vi "Generate SBOM from VIPC.vi"() -> ()   [LabVIEW 2017]
uses:
  <vilib>/JKI/VIPM API/command-line/support/Library Contents Cluster_vipm_api.ctl
  <vilib>/JKI/VIPM API/VIPM API_vipm_api.lvlib
  VIP Support/VIP SBOM Support.lvlib
panel:
  in  "VIPC File Path":path
  out "SBOM":string[][](table)
  out "CSV SBOM":string
  out "Packages in VIPC":T1[](array[typedef])
  # "Retrieves package information from the specified VIPC file"
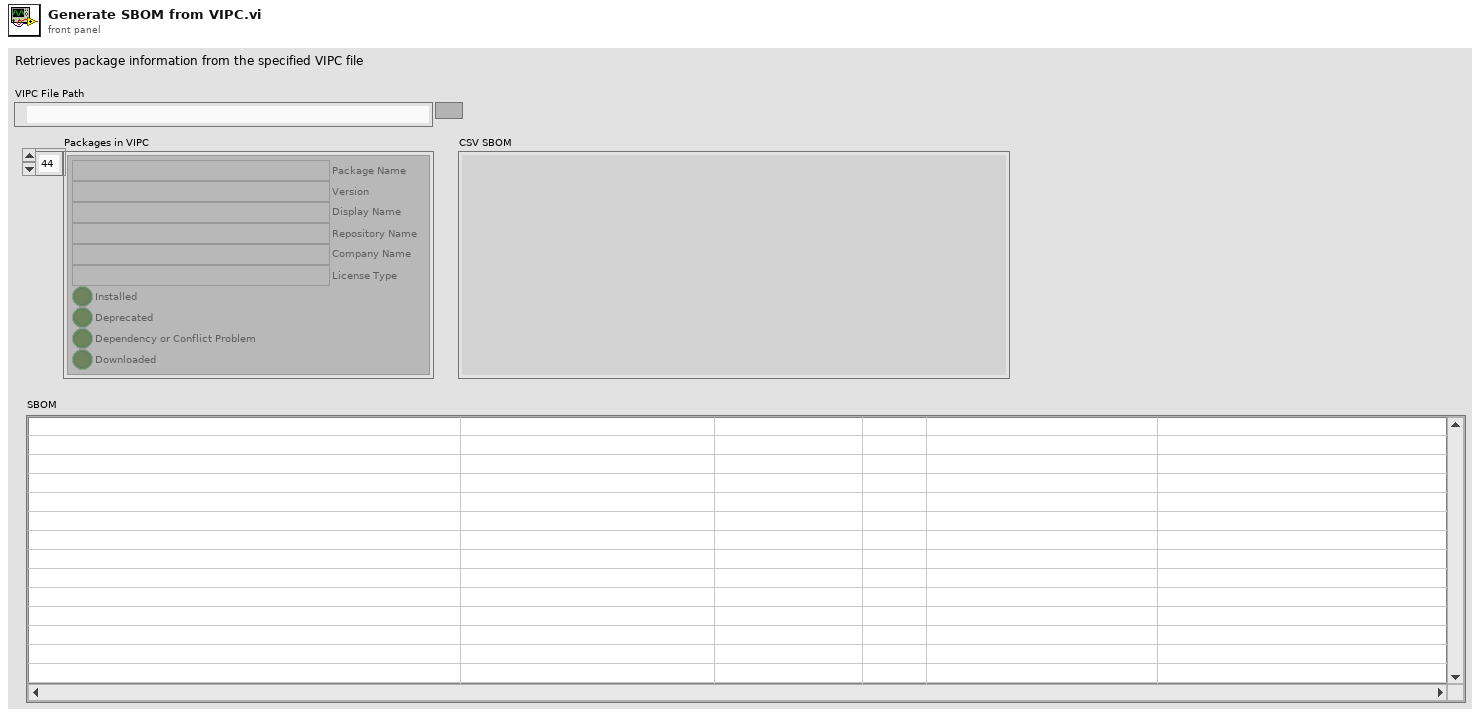
[diagram p1: front panel]
types:
  T1 = typedef "VIPM API_vipm_api.lvlib/Library Contents Cluster_vipm_api.ctl" = cluster{"Package Name":string, "Version":string, "Display Name":string, "Repository Name":string, "Company Name":string, "License Type":string, "Installed":bool, "Deprecated":bool, "Dependency or Conflict Problem":bool, "Downloaded":bool}
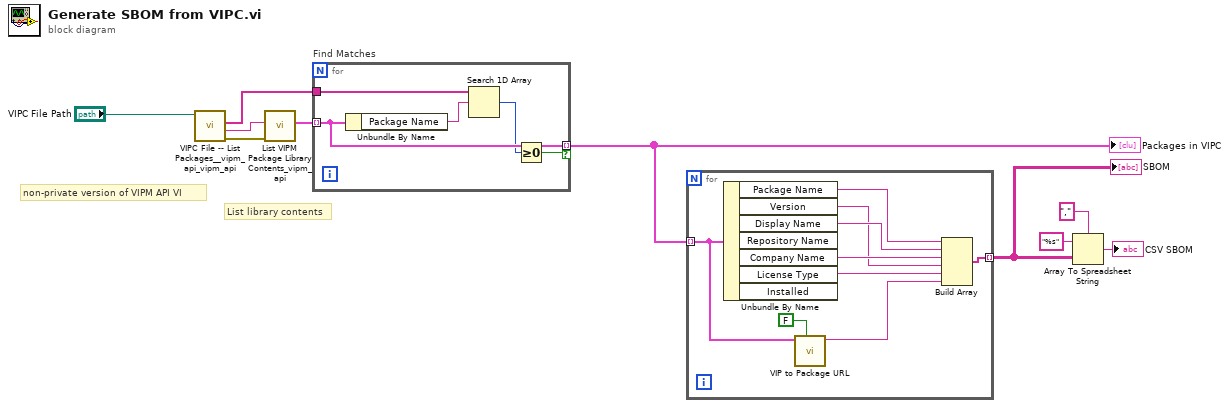
[diagram p0: block diagram]
diagram:
  # "List library contents"
  # "non-private version of VIPM API VI"
  n1 = call "VIPC File -- List Packages__vipm_api_vipm_api.vi"("VIPC File Path"="VIPC File Path") -> ("error out"=w3:errorcluster, "VIPC LabVIEW Version"=w1:string, "Package List"=w2:string[])  [unwired: 7 in, 1 out]
  n2 = call <vilib>:"List VIPM Package Library Contents_vipm_api.vi"("error in (no error)"=w3, "LabVIEW Version"=w1) -> ("Library Contents []"=w5:T1[])  [unwired: 8 in, 1 out]
  n3 = for "Find Matches" {
    tunnel: w5 -> [w15] mode=indexing
    tunnel: w2 -> [w14]
    tunnel: [w15] -> w10 mode=indexing if=w12
    n4 = Unbundle By Name(w15) -> ("Package Name"=w13:string)
    n5 = Search 1D Array(1D array=w14, element=w13) -> (index of element=w11:i32)  [unwired: 1 in]
    n6 = Greater Or Equal To 0?(x=w11) -> (x >= 0?=w12:bool)
  }
  "Packages in VIPC" <- w10
  n7 = for {
    tunnel: w10 -> [w18] mode=indexing
    tunnel: [w19] -> w6 mode=indexing
    n8 = Unbundle By Name(w18) -> ("Package Name"=w24:string, "Version"=w21:string, "Display Name"=w23:string, "Company Name"=w22:string, "License Type"=w20:string)  [unwired: 2 out]
    n9 = call "VIP to Package URL.vi"("Include Repository?"=FALSE ("Include Repositories?"), "VIP Information"=w18) -> ("VIP Package URL"=w17:string)  [unwired: 9 in]
    n10 = Build Array(w24, w23, w22, w21, w20, w17) -> (w19:string[])
  }
  "SBOM" <- w6
  n11 = Array To Spreadsheet String(delimiter (Tab)=",", array=w6, 3:"%s" ("format string")) -> (spreadsheet string=→"CSV SBOM":string)
